vi "Connect.vi"(8 "error in (no error)":errorcluster, 11 "Serial Device in":refnum<class "Serial Device.lvclass">) -> (0 "error out":errorcluster, 3 "Serial Device out":refnum<class "Serial Device.lvclass">)   [LabVIEW 2017, in "Serial Device.lvclass"]
uses:
  Serial Device.lvclass
  Serial Device.lvclass/Serial Device.ctl
  Get Serial Port.vi
  Set Serial Port.vi
  <vilib>/Instr/_visa.llb/VISA Configure Serial Port (Instr).vi
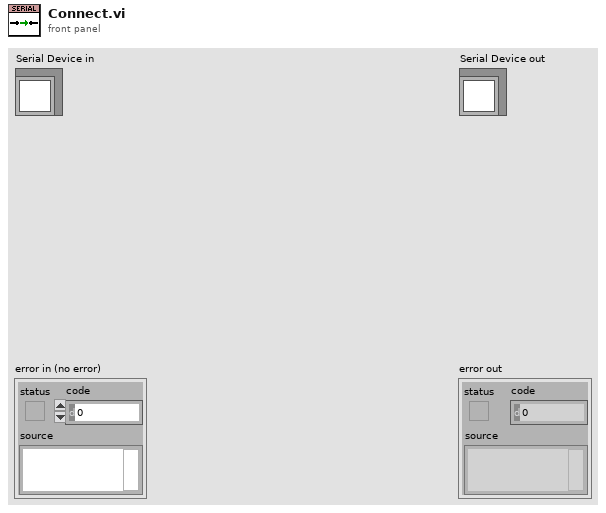
[diagram p1: front panel]
types:
  T1 = typedef "Serial Port configuration--cluster.ctl" = cluster{"Port":refnum<visa-resource-name>, "Bits per second (baud rate)":u32, "Data bits":u16, "Parity":enum16{"None", "Odd", "Even", "Mark", "Space"}, "Stop bits":u16, "Flow control":u16, "Timeout (seconds)":u32, "Delay before read":dbl, "Termination Character":string, "Enable Termination Character":bool}
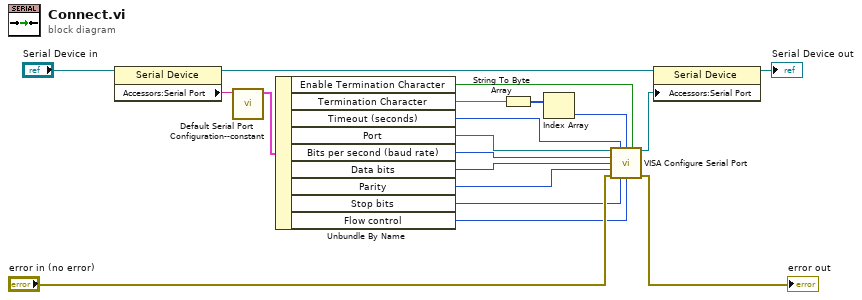
[diagram p0: block diagram]
diagram:
  n1 = property on="Property Node" class="Serial Device"(reference="Serial Device in") -> (reference out=w17:refnum<class "Serial Device.lvclass">, "Accessors:Serial Port"=w13:string)  [unwired: 1 in, 1 out]
  n2 = call "Default Serial Port Configuration--constant.vi"("Port"=w13) -> ("Serial Port Config"=w12:T1)  [unwired: 10 in]
  n3 = Unbundle By Name(w12) -> ("Enable Termination Character"=w6:bool, "Termination Character"=w9:string, "Timeout (seconds)"=w10:u32, "Port"=w11:refnum<visa-resource-name>, "Bits per second (baud rate)"=w5:u32, "Data bits"=w4:u16, "Parity"=w3:enum16{"None", "Odd", "Even", "Mark", "Space"}, "Stop bits"=w2:u16, "Flow control"=w1:u16)
  n4 = String To Byte Array(string=w9) -> (unsigned byte array=w8:u8[])
  n5 = Index Array(array=w8) -> (element=w7:u8)  [unwired: 1 in]
  n6 = call-poly "VISA Configure Serial Port"("VISA resource name"=w11, "timeout (10sec)"=w10, "termination char\n(0xA = '\\n' = LF)"=w7, "Enable Termination\nChar (T)"=w6, "baud rate (9600)"=w5, "data bits (8)"=w4, "parity (0:none)"=w3, "error in (no error)"="error in (no error)", "stop bits (10: 1 bit)"=w2, "flow control (0:none)"=w1) -> ("VISA resource name out"=w14:refnum<visa-resource-name>, "error out"=→"error out":errorcluster)  [unwired: 4 in]
  n7 = property on="Property Node" class="Serial Device"(reference=w17, "Accessors:Serial Port"=w14) -> (reference out=→"Serial Device out":refnum<class "Serial Device.lvclass">)  [unwired: 1 in, 1 out]
